vi "Employee Salary Info to Variant Array.vi"(8 "error in (no error)":errorcluster caption="错误输入（无错误）", 10 "Salary Info":T1, 11 "Employee 输入":refnum<class "Employee.lvclass"> caption="DNL_LabVIEW Object in") -> (0 "error out":errorcluster caption="错误输出", 2 "Salary Variant Array":variant[](array[variant]), 3 "Employee 输出":refnum<class "Employee.lvclass"> caption="DNL_LabVIEW Object out")   [LabVIEW 2012, in "Employee.lvclass"]
uses:
  Employee.lvclass
  Custom Def/Salary Info.ctl
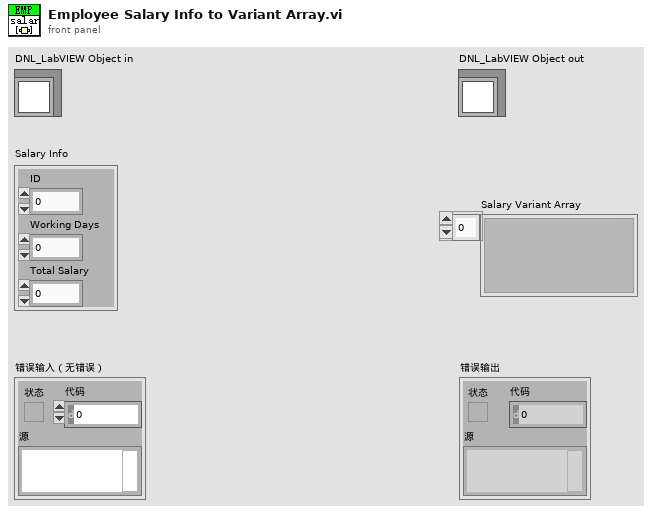
[diagram p1: front panel]
types:
  T1 = typedef "Salary Info.ctl" = cluster{"ID":u16, "Working Days":dbl, "Total Salary":dbl}
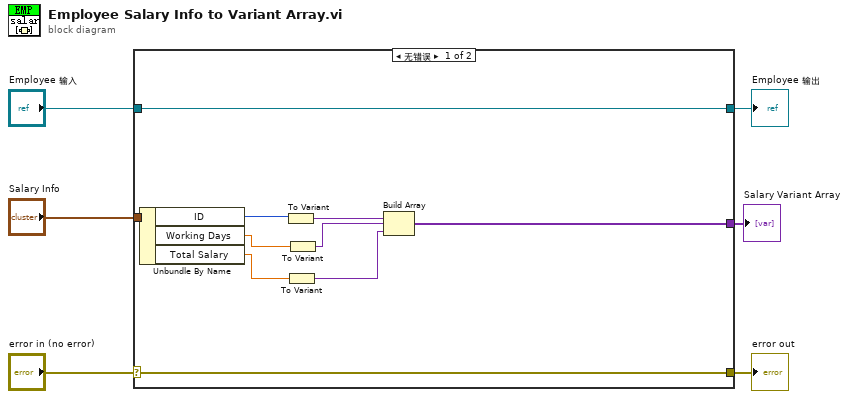
[diagram p0: block diagram]
diagram:
  n1 = case shown="无错误" "error in (no error)" {
    selector: "error in (no error)" -> [w15 w18]
    tunnel: [w15 w18] -> w5
    tunnel: [w16 w17] -> w3
    tunnel: "Employee 输入" -> [w16 w17]
    tunnel: "Salary Info" -> [w14 _]
    tunnel: [w7 _] -> w1
    frame No Error {
      n2 = Unbundle By Name(w14) -> ("ID"=w13:u16, "Working Days"=w12:dbl, "Total Salary"=w11:dbl)
      n3 = To Variant(anything=w13) -> (Variant=w10:variant)
      n4 = To Variant(anything=w11) -> (Variant=w8:variant)
      n5 = To Variant(anything=w12) -> (Variant=w9:variant)
      n6 = Build Array(w10, w9, w8) -> (w7:variant[])
    }
    frame Error {
    }
  }
  "error out" <- w5
  "Employee 输出" <- w3
  "Salary Variant Array" <- w1
